vi "Call Subpanel VI.vi"(8 "error in (no error)":errorcluster, 10 "VI Refnum":refnum<vi>, 11 "MotionSystem Configuration in":refnum<class "MotionSystem Configuration.lvclass">) -> (0 "error out":errorcluster, 3 "MotionSystem Configuration out":refnum<class "MotionSystem Configuration.lvclass">)   [LabVIEW 2016, in "MotionSystem.lvlib" / "MotionSystem Configuration.lvclass"]
uses:
  <userlib>/Common Components/Hardware/Abstract System/MotionSystem/MotionSystem Config/MotionSystem Configuration.lvclass
  <userlib>/Configuration Dialog Actor/Configuration.lvclass
  C:/Program Files (x86)/National Instruments/LabVIEW 2016/user.lib/Configuration Dialog Actor/Configuration.lvclass
  <userlib>/Configuration Dialog Actor/Configuration.lvclass/Configuration.ctl
  <userlib>/Common Components/Hardware/Abstract System/MotionSystem/MotionSystem Config/MotionSystem Configuration.lvclass/MotionSystem Configuration.ctl
  <userlib>/Common Components/Hardware/Abstract System/MotionSystem/MotionSystem Config/Accessors/Write Array of Motor Configuration Objs.vi
  <userlib>/Common Components/Hardware/Abstract System/MotionSystem/MotionSystem Config/Accessors/Read MotionSystem Obj.vi
  <userlib>/Common Components/Hardware/Abstract System/MotionSystem/MotionSystem Config/Accessors/Write MotionSystem Obj.vi
  <userlib>/Common Components/Hardware/Abstract System/MotionSystem/MotionSystem Config/Accessors/Read Array of Motor Category Strings.vi
  <userlib>/Common Components/Hardware/Abstract System/MotionSystem/MotionSystem Config/Accessors/Read Array of Motor Configuration Objs.vi
  <userlib>/Common Components/Hardware/Motor/Motor Config/Accessors/Read Motor Obj.vi
  <userlib>/Common Components/Hardware/Abstract System/MotionSystem/MotionSystem/MotionSystem.lvclass
  <userlib>/Common Components/Hardware/Motor/Motor/Motor.lvclass
  <userlib>/Common Components/Hardware/Motor/Motor Config/Motor Configuration.lvclass
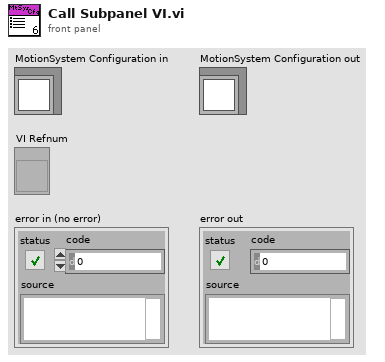
[diagram p1: front panel]
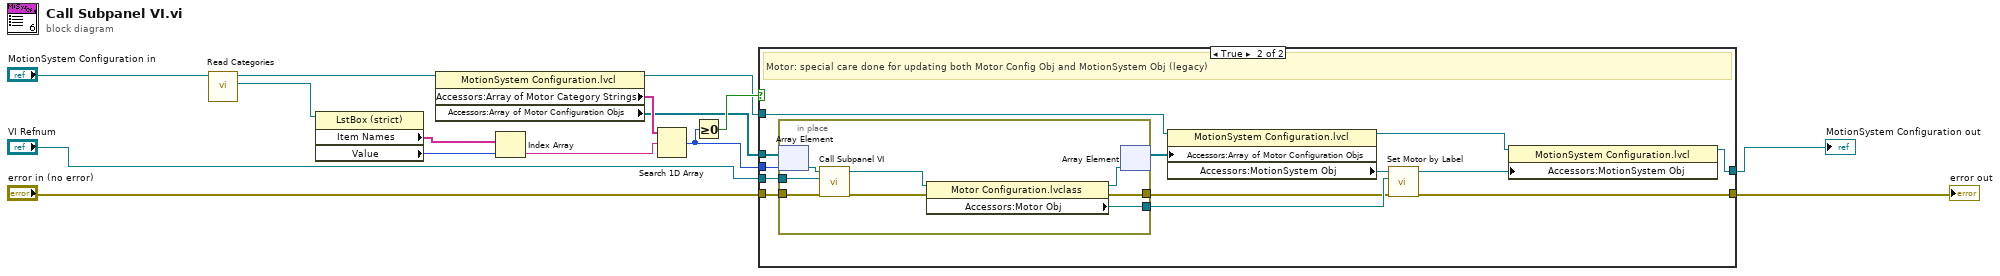
[diagram p0: block diagram]
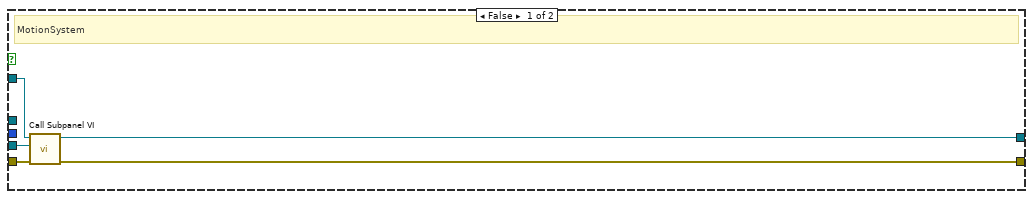
[diagram p2: hidden frame]
diagram:
  n1 = call <userlib>:"Read Categories.vi"("Configuration in"="MotionSystem Configuration in") -> ("Categories"=w11:refnum<vi>, "Configuration out"=w12:refnum<class "MotionSystem Configuration.lvclass">)  [unwired: 8 in, 1 out]
  n2 = property class="LstBox (strict)"(reference=w11) -> ("Item Names"=w10:string[], "Value"=w9:i32)  [unwired: 1 in, 2 out]
  n3 = property class="MotionSystem Configuration.lvcl"(reference=w12) -> (reference out=w1:refnum<class "MotionSystem Configuration.lvclass">, "Accessors:Array of Motor Category Strings"=w8:string[], "Accessors:Array of Motor Configuration Objs"=w5:refnum<class "Motor Configuration.lvclass">[])  [unwired: 1 in, 1 out]
  n4 = Index Array(array=w10, index=w9) -> (element=w7:string)
  n5 = Search 1D Array(1D array=w8, element=w7) -> (index of element=w4:i32)  [unwired: 1 in]
  n6 = Greater Or Equal To 0?(x=w4) -> (x >= 0?=w6:bool)
  n7 = case shown="True" w6 {
    tunnel: [w16 w21] -> w3
    tunnel: [w19 w23] -> w2
    tunnel: "error in (no error)" -> [w18 w33]
    tunnel: "VI Refnum" -> [w17 w32]
    tunnel: w1 -> [w20 w29]
    tunnel: w5 -> [_ w31]
    tunnel: w4 -> [_ w30]
    frame False {
      # "MotionSystem"
      n8 = call-parent "Call Subpanel VI.vi"("error in (no error)"=w18, "VI Refnum"=w17, "Configuration in"=w20) -> ("error out"=w16:errorcluster, "Configuration out"=w19:refnum<class "MotionSystem Configuration.lvclass">)  [unwired: 7 in]
    }
    frame True {
      # "Motor: special care done for updating both Motor Config Obj and MotionSystem Obj (legacy)"
      n9 = in-place {
        in-place-border: [w39] -> w22
        in-place-border: w33 -> [w41]
        in-place-border: w32 -> [w34]
        in-place-border: [w40] -> w26
        n10 = in-place-array #1(w31, w30) -> (w38:refnum<class "Motor Configuration.lvclass">)
        n11 = call-dynamic "Call Subpanel VI.vi"("error in (no error)"=w41, "VI Refnum"=w34, "Motor Configuration in"=w38) -> ("error out"=w37:errorcluster, "Motor Configuration out"=w36:refnum<class "Motor Configuration.lvclass">)  [unwired: 7 in]
        n12 = property class="Motor Configuration.lvclass"(reference=w36, error in=w37) -> (reference out=w35:refnum<class "Motor Configuration.lvclass">, error out=w39:errorcluster, "Accessors:Motor Obj"=w40:refnum<class "Motor.lvclass">)
        n13 = in-place-array #1(w35) -> (w28:refnum<class "Motor Configuration.lvclass">[])  [unwired: 1 out]
      }
      n14 = property class="MotionSystem Configuration.lvcl"(reference=w29, "Accessors:Array of Motor Configuration Objs"=w28) -> (reference out=w25:refnum<class "MotionSystem Configuration.lvclass">, "Accessors:MotionSystem Obj"=w27:refnum<class "MotionSystem.lvclass">)  [unwired: 1 in, 1 out]
      n15 = call <userlib>:"Set Motor by Label.vi"("error in (no error)"=w22, "Motor obj"=w26, "MotionSystem in"=w27) -> ("error out"=w21:errorcluster, "MotionSystem out"=w24:refnum<class "MotionSystem.lvclass">)  [unwired: 7 in]
      n16 = property class="MotionSystem Configuration.lvcl"(reference=w25, "Accessors:MotionSystem Obj"=w24) -> (reference out=w23:refnum<class "MotionSystem Configuration.lvclass">)  [unwired: 1 in, 1 out]
    }
  }
  "error out" <- w3
  "MotionSystem Configuration out" <- w2
